vi "Serial Convert.vi"(8 "Range (V)":sgl=20.0 format="%#_13g", 10 "N channels bytes to read":u8=18, 11 "Raw serial buffer":string="\u0000\u0000\u0000\u0000\u0000\u0000\u0000\u0000\u0000\u0000\u0000\u0000\u0000\u0000\u0000\u0000\u0000\u0000") -> (0 "V6 (V)":sgl, 1 "V5 (V)":sgl, 2 "V4 (V)":sgl, 3 "V3 (V)":sgl, 4 "V7 (V)":sgl, 5 "V2 (V)":sgl, 6 "V8 (V)":sgl, 7 "V1 (V)":sgl)   [LabVIEW 2015]
panel:
  # "PN 19/12/2014, 17/08/2015 (nChan optimisation)"
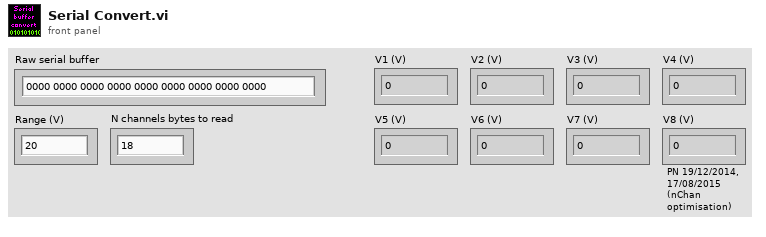
[diagram p1: front panel]
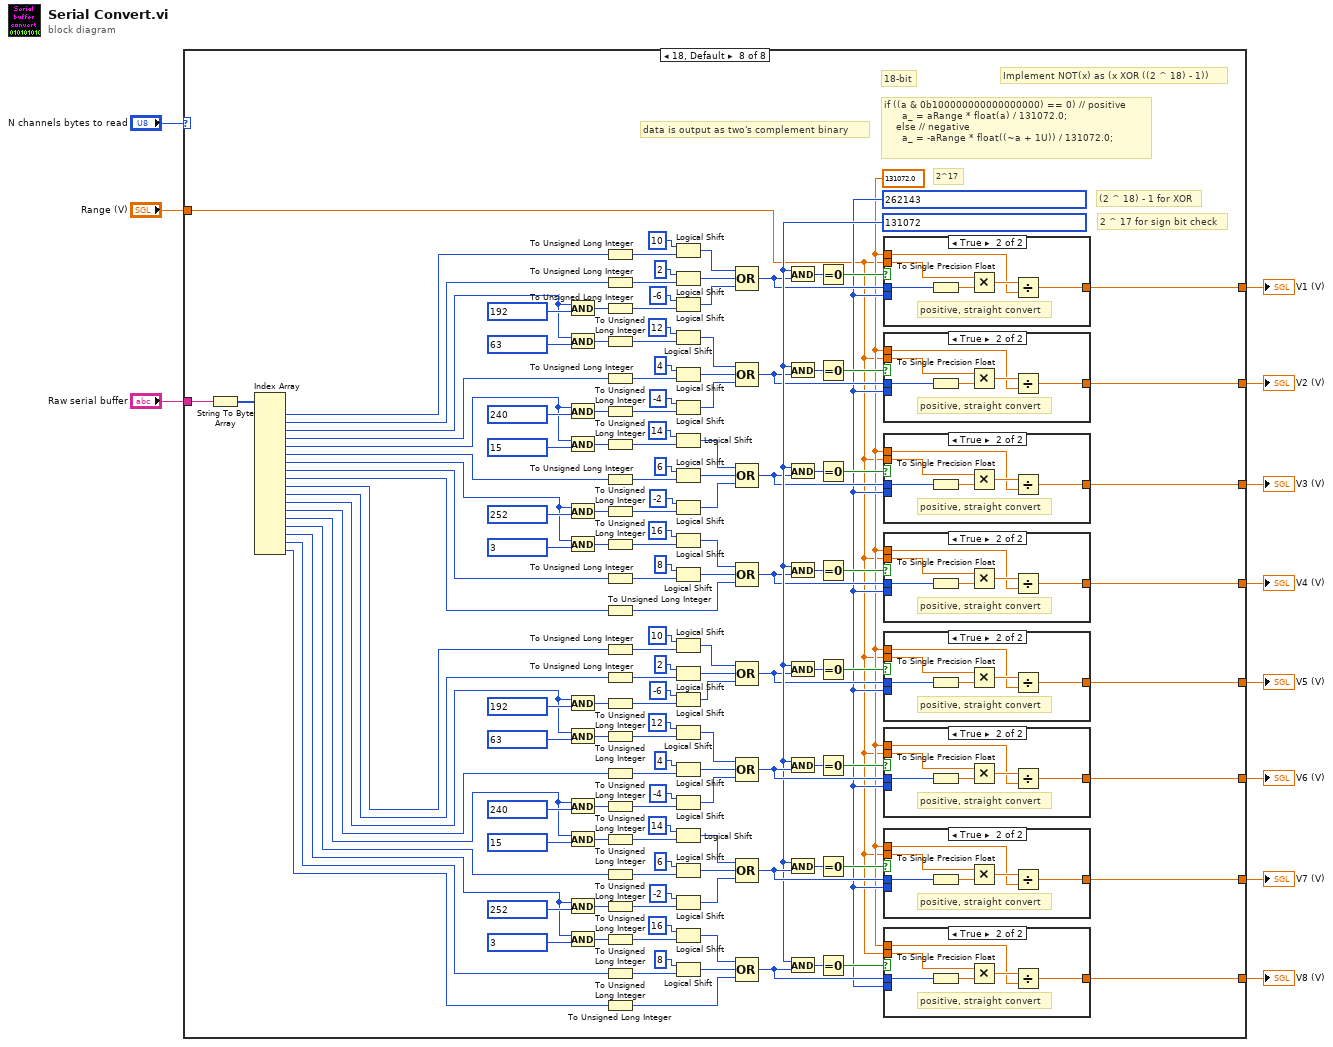
[diagram p0: block diagram]
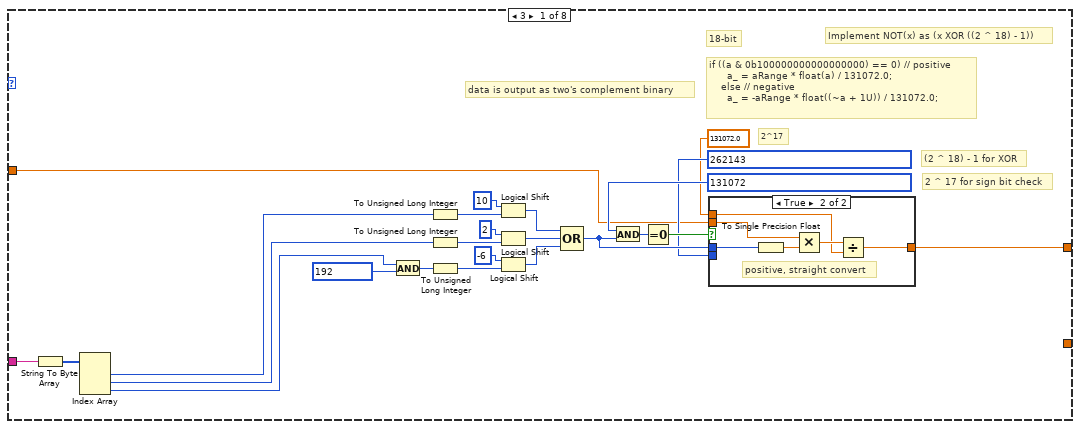
[diagram p2: hidden frame]
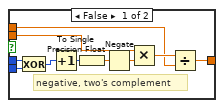
[diagram p3: hidden frame]
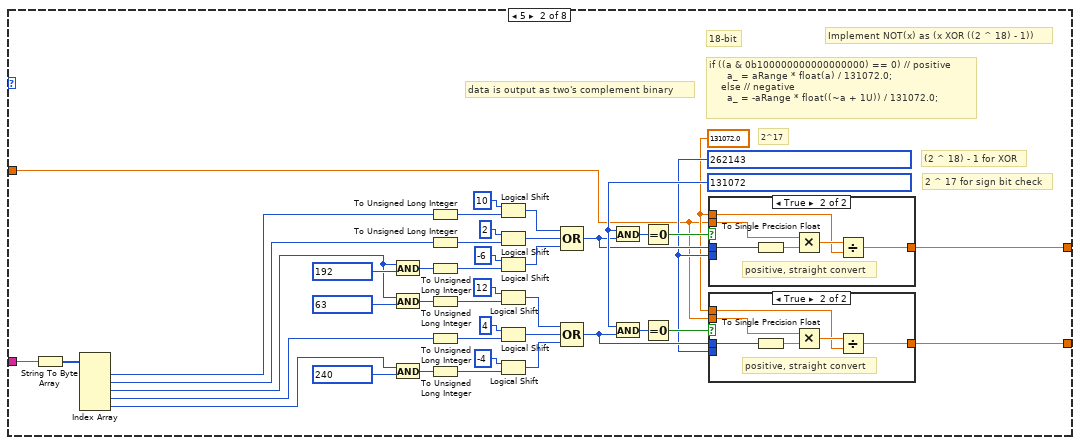
[diagram p4: hidden frame]
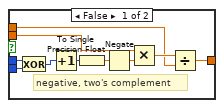
[diagram p5: hidden frame]
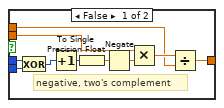
[diagram p6: hidden frame]
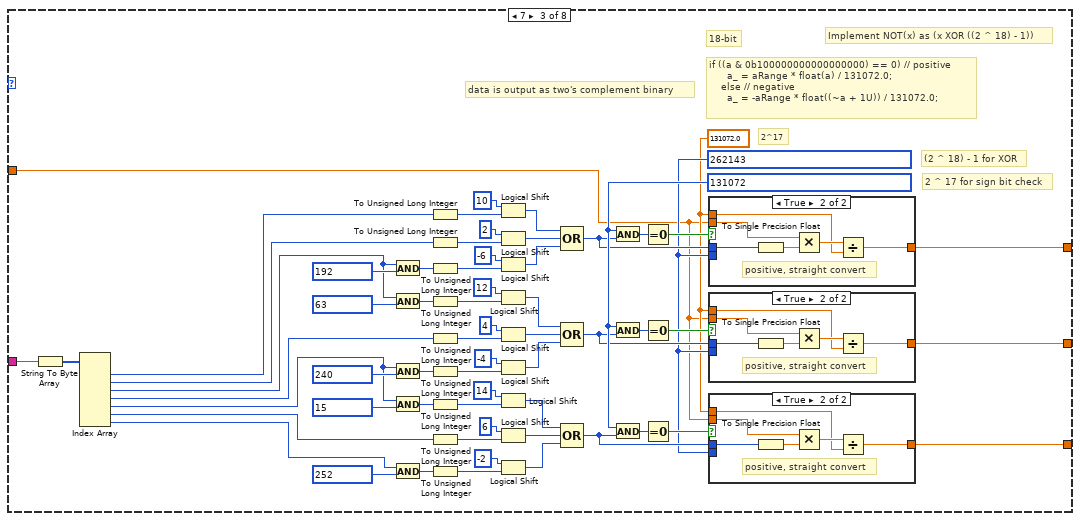
[diagram p7: hidden frame]
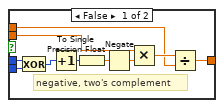
[diagram p8: hidden frame]
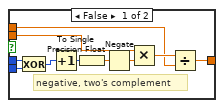
[diagram p9: hidden frame]
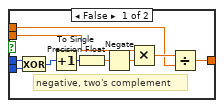
[diagram p10: hidden frame]
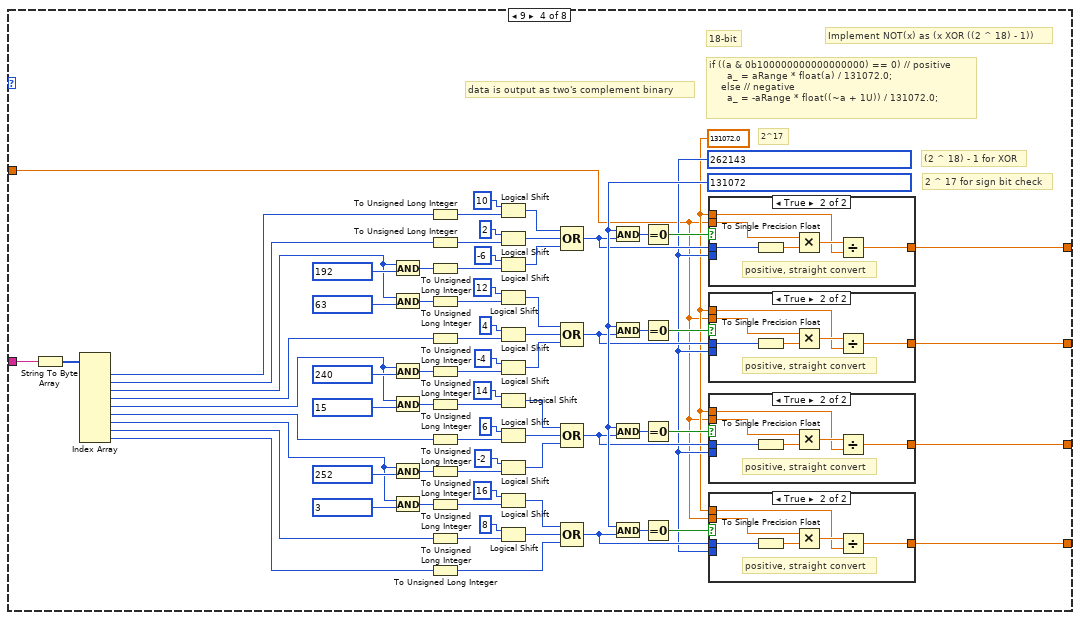
[diagram p11: hidden frame]
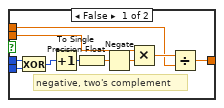
[diagram p12: hidden frame]
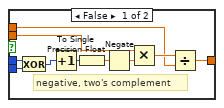
[diagram p13: hidden frame]
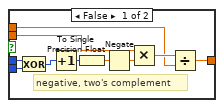
[diagram p14: hidden frame]
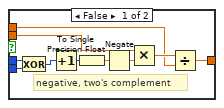
[diagram p15: hidden frame]
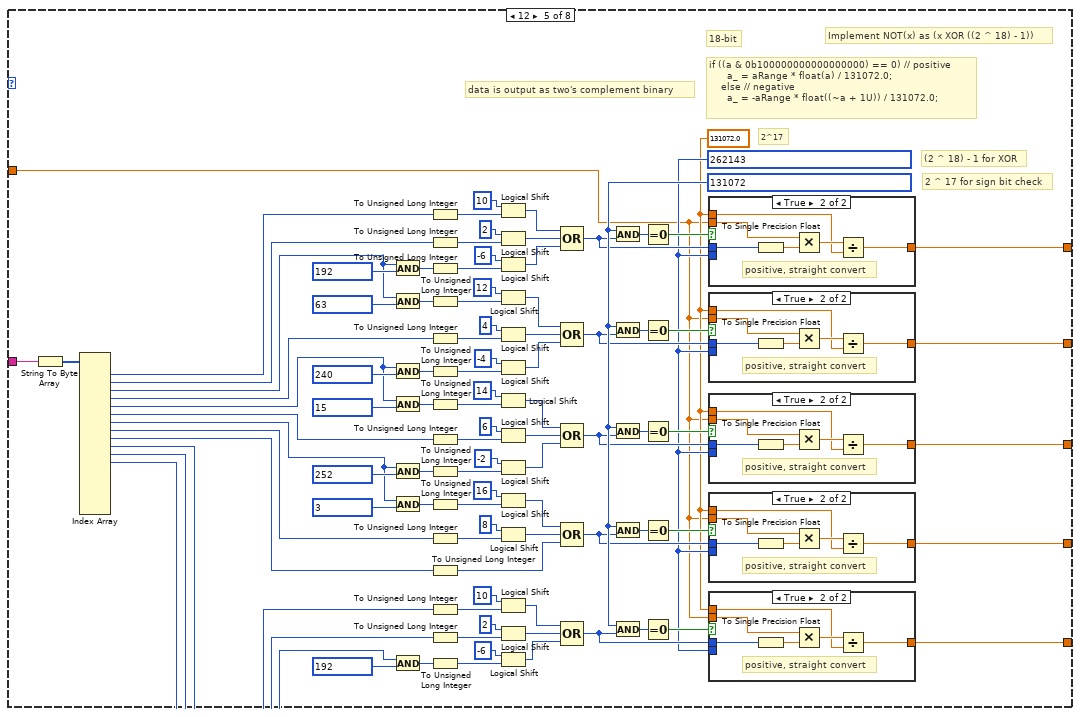
[diagram p16: hidden frame]
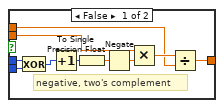
[diagram p17: hidden frame]
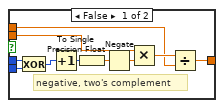
[diagram p18: hidden frame]
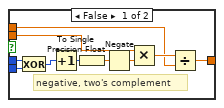
[diagram p19: hidden frame]
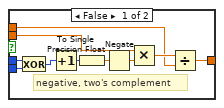
[diagram p20: hidden frame]
diagram:
  n1 = case shown="18, Default" "N channels bytes to read" {
    tunnel: "Raw serial buffer" -> [w35 w94 w188 w313 w472 w666 w895 w1155]
    tunnel: [_ _ _ _ _ _ w841 w1100] -> w10
    tunnel: [_ _ _ _ _ w613 w840 w1099] -> w9
    tunnel: [_ _ _ _ _ _ _ w1044] -> w8
    tunnel: [w20 w66 w147 w260 w407 w585 w798 w1043] -> w7
    tunnel: [_ _ w143 w256 w403 w581 w794 w1039] -> w6
    tunnel: [_ w63 w142 w255 w402 w580 w793 w1038] -> w5
    tunnel: [_ _ _ w254 w401 w579 w792 w1037] -> w4
    tunnel: [_ _ _ _ w400 w578 w791 w1036] -> w3
    tunnel: "Range (V)" -> [w15 w58 w136 w246 w390 w568 w781 w1026]
    frame 3 {
      # "2 ^ 17 for sign bit check"
      # "(2 ^ 18) - 1 for XOR"
      # "Implement NOT(x) as (x XOR ((2 ^ 18) - 1))"
      # "18-bit"
      # "2^17"
      # "data is output as two's complement binary"
      # "if ((a & 0b100000000000000000) == 0) // positive\n      a_ = aRange * float(a) / 131072.0; \n    else // negative\n      a_ = -aRange * float((~a + 1U)) / 131072.0;"
      n2 = String To Byte Array(string=w35) -> (unsigned byte array=w30:u8[])
      n3 = Index Array(array=w30) -> (element #1=w34:u8, element #2=w31:u8, element #3=w23:u8)  [unwired: 3 in]
      n4 = And(x=w23, y=u8 192) -> (x .and. y?=w26:u8)
      n5 = To Unsigned Long Integer(number=w34) -> (unsigned 32bit integer=w29:u32)
      n6 = To Unsigned Long Integer(number=w31) -> (unsigned 32bit integer=w28:u32)
      n7 = To Unsigned Long Integer(number=w26) -> (unsigned 32bit integer=w13:u32)
      n8 = Logical Shift(y=i16 10, x=w29) -> (x << y=w24:u32)
      n9 = Logical Shift(y=i16 2, x=w28) -> (x << y=w25:u32)
      n10 = Logical Shift(y=i16 -6, x=w13) -> (x << y=w12:u32)
      n11 = Compound Arithmetic op=OR(w24, w25, w12) -> (w18:u32)
      n12 = And(x=u32 131072, y=w18) -> (x .and. y?=w22:u32)
      n13 = Equal To 0?(x=w22) -> (x = 0?=w19:bool)
      n14 = case shown="True" w19 {
        tunnel: w15 -> [w42 w49]
        tunnel: sgl 131072.0 -> [w41 w47]
        tunnel: w18 -> [w37 w51]
        tunnel: [w40 w46] -> w20
        tunnel: u32 262143 -> [w36 _]
        frame False {
          # "negative, two's complement"
          n15 = Exclusive Or(1:w36, 2:w37) -> (0:w38:u32)
          n16 = Increment(x=w38) -> (x+1=w43:u32)
          n17 = To Single Precision Float(number=w43) -> (single precision float=w45:sgl)
          n18 = Negate(x=w45) -> (-x=w39:sgl)
          n19 = Multiply(x=w42, y=w39) -> (x*y=w44:sgl)
          n20 = Divide(x=w44, y=w41) -> (x/y=w40:sgl)
        }
        frame True {
          # "positive, straight convert"
          n21 = To Single Precision Float(number=w51) -> (single precision float=w50:sgl)
          n22 = Multiply(x=w49, y=w50) -> (x*y=w48:sgl)
          n23 = Divide(x=w48, y=w47) -> (x/y=w46:sgl)
        }
      }
    }
    frame 5 {
      w60 = u32 262143
      w59 = sgl 131072.0
      w67 = u32 131072
      # "2 ^ 17 for sign bit check"
      # "(2 ^ 18) - 1 for XOR"
      # "Implement NOT(x) as (x XOR ((2 ^ 18) - 1))"
      # "18-bit"
      # "2^17"
      # "data is output as two's complement binary"
      # "if ((a & 0b100000000000000000) == 0) // positive\n      a_ = aRange * float(a) / 131072.0; \n    else // negative\n      a_ = -aRange * float((~a + 1U)) / 131072.0;"
      n24 = String To Byte Array(string=w94) -> (unsigned byte array=w89:u8[])
      n25 = Index Array(array=w89) -> (element #1=w93:u8, element #2=w90:u8, element #3=w81:u8, element #4=w77:u8, element #5=w70:u8)  [unwired: 5 in]
      n26 = And(x=w81, y=u8 192) -> (x .and. y?=w85:u8)
      n27 = And(x=w81, y=u8 63) -> (x .and. y?=w80:u8)
      n28 = And(x=w70, y=u8 240) -> (x .and. y?=w73:u8)
      n29 = To Unsigned Long Integer(number=w93) -> (unsigned 32bit integer=w88:u32)
      n30 = To Unsigned Long Integer(number=w90) -> (unsigned 32bit integer=w87:u32)
      n31 = To Unsigned Long Integer(number=w85) -> (unsigned 32bit integer=w56:u32)
      n32 = To Unsigned Long Integer(number=w80) -> (unsigned 32bit integer=w79:u32)
      n33 = To Unsigned Long Integer(number=w77) -> (unsigned 32bit integer=w76:u32)
      n34 = To Unsigned Long Integer(number=w73) -> (unsigned 32bit integer=w53:u32)
      n35 = Logical Shift(y=i16 10, x=w88) -> (x << y=w83:u32)
      n36 = Logical Shift(y=i16 2, x=w87) -> (x << y=w84:u32)
      n37 = Logical Shift(y=i16 -6, x=w56) -> (x << y=w55:u32)
      n38 = Logical Shift(y=i16 12, x=w79) -> (x << y=w72:u32)
      n39 = Logical Shift(y=i16 4, x=w76) -> (x << y=w71:u32)
      n40 = Logical Shift(y=i16 -4, x=w53) -> (x << y=w52:u32)
      n41 = Compound Arithmetic op=OR(w83, w84, w55) -> (w64:u32)
      n42 = Compound Arithmetic op=OR(w72, w71, w52) -> (w61:u32)
      n43 = And(x=w67, y=w64) -> (x .and. y?=w69:u32)
      n44 = And(x=w67, y=w61) -> (x .and. y?=w68:u32)
      n45 = Equal To 0?(x=w69) -> (x = 0?=w65:bool)
      n46 = Equal To 0?(x=w68) -> (x = 0?=w62:bool)
      n47 = case shown="True" w65 {
        tunnel: w58 -> [w101 w108]
        tunnel: w59 -> [w100 w106]
        tunnel: w64 -> [w96 w110]
        tunnel: [w99 w105] -> w66
        tunnel: w60 -> [w95 _]
        frame False {
          # "negative, two's complement"
          n48 = Exclusive Or(1:w95, 2:w96) -> (0:w97:u32)
          n49 = Increment(x=w97) -> (x+1=w102:u32)
          n50 = To Single Precision Float(number=w102) -> (single precision float=w104:sgl)
          n51 = Negate(x=w104) -> (-x=w98:sgl)
          n52 = Multiply(x=w101, y=w98) -> (x*y=w103:sgl)
          n53 = Divide(x=w103, y=w100) -> (x/y=w99:sgl)
        }
        frame True {
          # "positive, straight convert"
          n54 = To Single Precision Float(number=w110) -> (single precision float=w109:sgl)
          n55 = Multiply(x=w108, y=w109) -> (x*y=w107:sgl)
          n56 = Divide(x=w107, y=w106) -> (x/y=w105:sgl)
        }
      }
      n57 = case shown="True" w62 {
        tunnel: w58 -> [w117 w124]
        tunnel: w59 -> [w116 w122]
        tunnel: w61 -> [w112 w126]
        tunnel: [w115 w121] -> w63
        tunnel: w60 -> [w111 _]
        frame False {
          # "negative, two's complement"
          n58 = Exclusive Or(1:w111, 2:w112) -> (0:w113:u32)
          n59 = Increment(x=w113) -> (x+1=w118:u32)
          n60 = To Single Precision Float(number=w118) -> (single precision float=w120:sgl)
          n61 = Negate(x=w120) -> (-x=w114:sgl)
          n62 = Multiply(x=w117, y=w114) -> (x*y=w119:sgl)
          n63 = Divide(x=w119, y=w116) -> (x/y=w115:sgl)
        }
        frame True {
          # "positive, straight convert"
          n64 = To Single Precision Float(number=w126) -> (single precision float=w125:sgl)
          n65 = Multiply(x=w124, y=w125) -> (x*y=w123:sgl)
          n66 = Divide(x=w123, y=w122) -> (x/y=w121:sgl)
        }
      }
    }
    frame 7 {
      w138 = u32 262143
      w137 = sgl 131072.0
      w148 = u32 131072
      # "2 ^ 17 for sign bit check"
      # "(2 ^ 18) - 1 for XOR"
      # "Implement NOT(x) as (x XOR ((2 ^ 18) - 1))"
      # "18-bit"
      # "2^17"
      # "data is output as two's complement binary"
      # "if ((a & 0b100000000000000000) == 0) // positive\n      a_ = aRange * float(a) / 131072.0; \n    else // negative\n      a_ = -aRange * float((~a + 1U)) / 131072.0;"
      n67 = String To Byte Array(string=w188) -> (unsigned byte array=w183:u8[])
      n68 = Index Array(array=w183) -> (element #1=w187:u8, element #2=w184:u8, element #3=w175:u8, element #4=w171:u8, element #5=w163:u8, element #6=w158:u8, element #7=w152:u8)  [unwired: 7 in]
      n69 = And(x=w175, y=u8 192) -> (x .and. y?=w179:u8)
      n70 = And(x=w175, y=u8 63) -> (x .and. y?=w174:u8)
      n71 = And(x=w163, y=u8 240) -> (x .and. y?=w167:u8)
      n72 = And(x=w163, y=u8 15) -> (x .and. y?=w162:u8)
      n73 = And(x=w152, y=u8 252) -> (x .and. y?=w153:u8)
      n74 = To Unsigned Long Integer(number=w187) -> (unsigned 32bit integer=w182:u32)
      n75 = To Unsigned Long Integer(number=w184) -> (unsigned 32bit integer=w181:u32)
      n76 = To Unsigned Long Integer(number=w179) -> (unsigned 32bit integer=w134:u32)
      n77 = To Unsigned Long Integer(number=w174) -> (unsigned 32bit integer=w173:u32)
      n78 = To Unsigned Long Integer(number=w171) -> (unsigned 32bit integer=w170:u32)
      n79 = To Unsigned Long Integer(number=w167) -> (unsigned 32bit integer=w131:u32)
      n80 = To Unsigned Long Integer(number=w162) -> (unsigned 32bit integer=w160:u32)
      n81 = To Unsigned Long Integer(number=w158) -> (unsigned 32bit integer=w156:u32)
      n82 = To Unsigned Long Integer(number=w153) -> (unsigned 32bit integer=w127:u32)
      n83 = Logical Shift(y=i16 10, x=w182) -> (x << y=w177:u32)
      n84 = Logical Shift(y=i16 2, x=w181) -> (x << y=w178:u32)
      n85 = Logical Shift(y=i16 -6, x=w134) -> (x << y=w133:u32)
      n86 = Logical Shift(y=i16 12, x=w173) -> (x << y=w166:u32)
      n87 = Logical Shift(y=i16 4, x=w170) -> (x << y=w165:u32)
      n88 = Logical Shift(y=i16 -4, x=w131) -> (x << y=w130:u32)
      n89 = Logical Shift(y=i16 14, x=w160) -> (x << y=w159:u32)
      n90 = Logical Shift(y=i16 6, x=w156) -> (x << y=w155:u32)
      n91 = Logical Shift(y=i16 -2, x=w127) -> (x << y=w128:u32)
      n92 = Compound Arithmetic op=OR(w177, w178, w133) -> (w145:u32)
      n93 = Compound Arithmetic op=OR(w166, w165, w130) -> (w139:u32)
      n94 = Compound Arithmetic op=OR(w159, w155, w128) -> (w141:u32)
      n95 = And(x=w148, y=w145) -> (x .and. y?=w151:u32)
      n96 = And(x=w148, y=w139) -> (x .and. y?=w150:u32)
      n97 = And(x=w148, y=w141) -> (x .and. y?=w149:u32)
      n98 = Equal To 0?(x=w151) -> (x = 0?=w146:bool)
      n99 = Equal To 0?(x=w150) -> (x = 0?=w140:bool)
      n100 = Equal To 0?(x=w149) -> (x = 0?=w144:bool)
      n101 = case shown="True" w146 {
        tunnel: w136 -> [w195 w202]
        tunnel: w137 -> [w194 w200]
        tunnel: w145 -> [w190 w204]
        tunnel: [w193 w199] -> w147
        tunnel: w138 -> [w189 _]
        frame False {
          # "negative, two's complement"
          n102 = Exclusive Or(1:w189, 2:w190) -> (0:w191:u32)
          n103 = Increment(x=w191) -> (x+1=w196:u32)
          n104 = To Single Precision Float(number=w196) -> (single precision float=w198:sgl)
          n105 = Negate(x=w198) -> (-x=w192:sgl)
          n106 = Multiply(x=w195, y=w192) -> (x*y=w197:sgl)
          n107 = Divide(x=w197, y=w194) -> (x/y=w193:sgl)
        }
        frame True {
          # "positive, straight convert"
          n108 = To Single Precision Float(number=w204) -> (single precision float=w203:sgl)
          n109 = Multiply(x=w202, y=w203) -> (x*y=w201:sgl)
          n110 = Divide(x=w201, y=w200) -> (x/y=w199:sgl)
        }
      }
      n111 = case shown="True" w140 {
        tunnel: w136 -> [w211 w218]
        tunnel: w137 -> [w210 w216]
        tunnel: w139 -> [w206 w220]
        tunnel: [w209 w215] -> w142
        tunnel: w138 -> [w205 _]
        frame False {
          # "negative, two's complement"
          n112 = Exclusive Or(1:w205, 2:w206) -> (0:w207:u32)
          n113 = Increment(x=w207) -> (x+1=w212:u32)
          n114 = To Single Precision Float(number=w212) -> (single precision float=w214:sgl)
          n115 = Negate(x=w214) -> (-x=w208:sgl)
          n116 = Multiply(x=w211, y=w208) -> (x*y=w213:sgl)
          n117 = Divide(x=w213, y=w210) -> (x/y=w209:sgl)
        }
        frame True {
          # "positive, straight convert"
          n118 = To Single Precision Float(number=w220) -> (single precision float=w219:sgl)
          n119 = Multiply(x=w218, y=w219) -> (x*y=w217:sgl)
          n120 = Divide(x=w217, y=w216) -> (x/y=w215:sgl)
        }
      }
      n121 = case shown="True" w144 {
        tunnel: w136 -> [w227 w234]
        tunnel: w137 -> [w226 w232]
        tunnel: w141 -> [w222 w236]
        tunnel: [w225 w231] -> w143
        tunnel: w138 -> [w221 _]
        frame False {
          # "negative, two's complement"
          n122 = Exclusive Or(1:w221, 2:w222) -> (0:w223:u32)
          n123 = Increment(x=w223) -> (x+1=w228:u32)
          n124 = To Single Precision Float(number=w228) -> (single precision float=w230:sgl)
          n125 = Negate(x=w230) -> (-x=w224:sgl)
          n126 = Multiply(x=w227, y=w224) -> (x*y=w229:sgl)
          n127 = Divide(x=w229, y=w226) -> (x/y=w225:sgl)
        }
        frame True {
          # "positive, straight convert"
          n128 = To Single Precision Float(number=w236) -> (single precision float=w235:sgl)
          n129 = Multiply(x=w234, y=w235) -> (x*y=w233:sgl)
          n130 = Divide(x=w233, y=w232) -> (x/y=w231:sgl)
        }
      }
    }
    frame 9 {
      w248 = u32 262143
      w247 = sgl 131072.0
      w261 = u32 131072
      # "2 ^ 17 for sign bit check"
      # "(2 ^ 18) - 1 for XOR"
      # "Implement NOT(x) as (x XOR ((2 ^ 18) - 1))"
      # "18-bit"
      # "2^17"
      # "data is output as two's complement binary"
      # "if ((a & 0b100000000000000000) == 0) // positive\n      a_ = aRange * float(a) / 131072.0; \n    else // negative\n      a_ = -aRange * float((~a + 1U)) / 131072.0;"
      n131 = String To Byte Array(string=w313) -> (unsigned byte array=w308:u8[])
      n132 = Index Array(array=w308) -> (element #1=w312:u8, element #2=w309:u8, element #3=w300:u8, element #4=w296:u8, element #5=w288:u8, element #6=w283:u8, element #7=w276:u8, element #8=w271:u8, element #9=w267:u8)  [unwired: 9 in]
      n133 = And(x=w300, y=u8 192) -> (x .and. y?=w304:u8)
      n134 = And(x=w300, y=u8 63) -> (x .and. y?=w299:u8)
      n135 = And(x=w288, y=u8 240) -> (x .and. y?=w292:u8)
      n136 = And(x=w288, y=u8 15) -> (x .and. y?=w287:u8)
      n137 = And(x=w276, y=u8 252) -> (x .and. y?=w278:u8)
      n138 = And(x=w276, y=u8 3) -> (x .and. y?=w275:u8)
      n139 = To Unsigned Long Integer(number=w312) -> (unsigned 32bit integer=w307:u32)
      n140 = To Unsigned Long Integer(number=w309) -> (unsigned 32bit integer=w306:u32)
      n141 = To Unsigned Long Integer(number=w304) -> (unsigned 32bit integer=w244:u32)
      n142 = To Unsigned Long Integer(number=w299) -> (unsigned 32bit integer=w298:u32)
      n143 = To Unsigned Long Integer(number=w296) -> (unsigned 32bit integer=w295:u32)
      n144 = To Unsigned Long Integer(number=w292) -> (unsigned 32bit integer=w241:u32)
      n145 = To Unsigned Long Integer(number=w287) -> (unsigned 32bit integer=w285:u32)
      n146 = To Unsigned Long Integer(number=w283) -> (unsigned 32bit integer=w281:u32)
      n147 = To Unsigned Long Integer(number=w278) -> (unsigned 32bit integer=w237:u32)
      n148 = To Unsigned Long Integer(number=w275) -> (unsigned 32bit integer=w273:u32)
      n149 = To Unsigned Long Integer(number=w271) -> (unsigned 32bit integer=w269:u32)
      n150 = To Unsigned Long Integer(number=w267) -> (unsigned 32bit integer=w266:u32)
      n151 = Logical Shift(y=i16 10, x=w307) -> (x << y=w302:u32)
      n152 = Logical Shift(y=i16 2, x=w306) -> (x << y=w303:u32)
      n153 = Logical Shift(y=i16 -6, x=w244) -> (x << y=w243:u32)
      n154 = Logical Shift(y=i16 12, x=w298) -> (x << y=w291:u32)
      n155 = Logical Shift(y=i16 4, x=w295) -> (x << y=w290:u32)
      n156 = Logical Shift(y=i16 -4, x=w241) -> (x << y=w240:u32)
      n157 = Logical Shift(y=i16 14, x=w285) -> (x << y=w284:u32)
      n158 = Logical Shift(y=i16 6, x=w281) -> (x << y=w280:u32)
      n159 = Logical Shift(y=i16 -2, x=w237) -> (x << y=w238:u32)
      n160 = Logical Shift(y=i16 16, x=w273) -> (x << y=w272:u32)
      n161 = Logical Shift(y=i16 8, x=w269) -> (x << y=w268:u32)
      n162 = Compound Arithmetic op=OR(w302, w303, w243) -> (w258:u32)
      n163 = Compound Arithmetic op=OR(w291, w290, w240) -> (w249:u32)
      n164 = Compound Arithmetic op=OR(w284, w280, w238) -> (w252:u32)
      n165 = Compound Arithmetic op=OR(w272, w268, w266) -> (w251:u32)
      n166 = And(x=w261, y=w258) -> (x .and. y?=w265:u32)
      n167 = And(x=w261, y=w249) -> (x .and. y?=w264:u32)
      n168 = And(x=w261, y=w252) -> (x .and. y?=w263:u32)
      n169 = And(x=w261, y=w251) -> (x .and. y?=w262:u32)
      n170 = Equal To 0?(x=w265) -> (x = 0?=w259:bool)
      n171 = Equal To 0?(x=w264) -> (x = 0?=w250:bool)
      n172 = Equal To 0?(x=w263) -> (x = 0?=w257:bool)
      n173 = Equal To 0?(x=w262) -> (x = 0?=w253:bool)
      n174 = case shown="True" w259 {
        tunnel: w246 -> [w320 w327]
        tunnel: w247 -> [w319 w325]
        tunnel: w258 -> [w315 w329]
        tunnel: [w318 w324] -> w260
        tunnel: w248 -> [w314 _]
        frame False {
          # "negative, two's complement"
          n175 = Exclusive Or(1:w314, 2:w315) -> (0:w316:u32)
          n176 = Increment(x=w316) -> (x+1=w321:u32)
          n177 = To Single Precision Float(number=w321) -> (single precision float=w323:sgl)
          n178 = Negate(x=w323) -> (-x=w317:sgl)
          n179 = Multiply(x=w320, y=w317) -> (x*y=w322:sgl)
          n180 = Divide(x=w322, y=w319) -> (x/y=w318:sgl)
        }
        frame True {
          # "positive, straight convert"
          n181 = To Single Precision Float(number=w329) -> (single precision float=w328:sgl)
          n182 = Multiply(x=w327, y=w328) -> (x*y=w326:sgl)
          n183 = Divide(x=w326, y=w325) -> (x/y=w324:sgl)
        }
      }
      n184 = case shown="True" w250 {
        tunnel: w246 -> [w336 w343]
        tunnel: w247 -> [w335 w341]
        tunnel: w249 -> [w331 w345]
        tunnel: [w334 w340] -> w255
        tunnel: w248 -> [w330 _]
        frame False {
          # "negative, two's complement"
          n185 = Exclusive Or(1:w330, 2:w331) -> (0:w332:u32)
          n186 = Increment(x=w332) -> (x+1=w337:u32)
          n187 = To Single Precision Float(number=w337) -> (single precision float=w339:sgl)
          n188 = Negate(x=w339) -> (-x=w333:sgl)
          n189 = Multiply(x=w336, y=w333) -> (x*y=w338:sgl)
          n190 = Divide(x=w338, y=w335) -> (x/y=w334:sgl)
        }
        frame True {
          # "positive, straight convert"
          n191 = To Single Precision Float(number=w345) -> (single precision float=w344:sgl)
          n192 = Multiply(x=w343, y=w344) -> (x*y=w342:sgl)
          n193 = Divide(x=w342, y=w341) -> (x/y=w340:sgl)
        }
      }
      n194 = case shown="True" w257 {
        tunnel: w246 -> [w352 w359]
        tunnel: w247 -> [w351 w357]
        tunnel: w252 -> [w347 w361]
        tunnel: [w350 w356] -> w256
        tunnel: w248 -> [w346 _]
        frame False {
          # "negative, two's complement"
          n195 = Exclusive Or(1:w346, 2:w347) -> (0:w348:u32)
          n196 = Increment(x=w348) -> (x+1=w353:u32)
          n197 = To Single Precision Float(number=w353) -> (single precision float=w355:sgl)
          n198 = Negate(x=w355) -> (-x=w349:sgl)
          n199 = Multiply(x=w352, y=w349) -> (x*y=w354:sgl)
          n200 = Divide(x=w354, y=w351) -> (x/y=w350:sgl)
        }
        frame True {
          # "positive, straight convert"
          n201 = To Single Precision Float(number=w361) -> (single precision float=w360:sgl)
          n202 = Multiply(x=w359, y=w360) -> (x*y=w358:sgl)
          n203 = Divide(x=w358, y=w357) -> (x/y=w356:sgl)
        }
      }
      n204 = case shown="True" w253 {
        tunnel: w246 -> [w368 w375]
        tunnel: w247 -> [w367 w373]
        tunnel: w251 -> [w363 w377]
        tunnel: [w366 w372] -> w254
        tunnel: w248 -> [w362 _]
        frame False {
          # "negative, two's complement"
          n205 = Exclusive Or(1:w362, 2:w363) -> (0:w364:u32)
          n206 = Increment(x=w364) -> (x+1=w369:u32)
          n207 = To Single Precision Float(number=w369) -> (single precision float=w371:sgl)
          n208 = Negate(x=w371) -> (-x=w365:sgl)
          n209 = Multiply(x=w368, y=w365) -> (x*y=w370:sgl)
          n210 = Divide(x=w370, y=w367) -> (x/y=w366:sgl)
        }
        frame True {
          # "positive, straight convert"
          n211 = To Single Precision Float(number=w377) -> (single precision float=w376:sgl)
          n212 = Multiply(x=w375, y=w376) -> (x*y=w374:sgl)
          n213 = Divide(x=w374, y=w373) -> (x/y=w372:sgl)
        }
      }
    }
    frame 12 {
      w392 = u32 262143
      w391 = sgl 131072.0
      w411 = u32 131072
      # "2 ^ 17 for sign bit check"
      # "(2 ^ 18) - 1 for XOR"
      # "Implement NOT(x) as (x XOR ((2 ^ 18) - 1))"
      # "18-bit"
      # "2^17"
      # "data is output as two's complement binary"
      # "if ((a & 0b100000000000000000) == 0) // positive\n      a_ = aRange * float(a) / 131072.0; \n    else // negative\n      a_ = -aRange * float((~a + 1U)) / 131072.0;"
      n214 = String To Byte Array(string=w472) -> (unsigned byte array=w467:u8[])
      n215 = Index Array(array=w467) -> (element #1=w471:u8, element #2=w468:u8, element #3=w459:u8, element #4=w455:u8, element #5=w447:u8, element #6=w442:u8, element #7=w435:u8, element #8=w430:u8, element #9=w426:u8, element #10=w410:u8, element #11=w409:u8, element #12=w408:u8)  [unwired: 18 in, 6 out]
      n216 = And(x=w459, y=u8 192) -> (x .and. y?=w463:u8)
      n217 = And(x=w459, y=u8 63) -> (x .and. y?=w458:u8)
      n218 = And(x=w447, y=u8 240) -> (x .and. y?=w451:u8)
      n219 = And(x=w447, y=u8 15) -> (x .and. y?=w446:u8)
      n220 = And(x=w435, y=u8 252) -> (x .and. y?=w437:u8)
      n221 = And(x=w435, y=u8 3) -> (x .and. y?=w434:u8)
      n222 = And(x=w408, y=u8 192) -> (x .and. y?=w417:u8)
      n223 = To Unsigned Long Integer(number=w471) -> (unsigned 32bit integer=w466:u32)
      n224 = To Unsigned Long Integer(number=w468) -> (unsigned 32bit integer=w465:u32)
      n225 = To Unsigned Long Integer(number=w463) -> (unsigned 32bit integer=w388:u32)
      n226 = To Unsigned Long Integer(number=w458) -> (unsigned 32bit integer=w457:u32)
      n227 = To Unsigned Long Integer(number=w455) -> (unsigned 32bit integer=w454:u32)
      n228 = To Unsigned Long Integer(number=w451) -> (unsigned 32bit integer=w382:u32)
      n229 = To Unsigned Long Integer(number=w446) -> (unsigned 32bit integer=w444:u32)
      n230 = To Unsigned Long Integer(number=w442) -> (unsigned 32bit integer=w440:u32)
      n231 = To Unsigned Long Integer(number=w437) -> (unsigned 32bit integer=w378:u32)
      n232 = To Unsigned Long Integer(number=w434) -> (unsigned 32bit integer=w432:u32)
      n233 = To Unsigned Long Integer(number=w430) -> (unsigned 32bit integer=w428:u32)
      n234 = To Unsigned Long Integer(number=w426) -> (unsigned 32bit integer=w425:u32)
      n235 = To Unsigned Long Integer(number=w410) -> (unsigned 32bit integer=w414:u32)
      n236 = To Unsigned Long Integer(number=w409) -> (unsigned 32bit integer=w415:u32)
      n237 = To Unsigned Long Integer(number=w417) -> (unsigned 32bit integer=w384:u32)
      n238 = Logical Shift(y=i16 10, x=w466) -> (x << y=w461:u32)
      n239 = Logical Shift(y=i16 2, x=w465) -> (x << y=w462:u32)
      n240 = Logical Shift(y=i16 -6, x=w388) -> (x << y=w387:u32)
      n241 = Logical Shift(y=i16 12, x=w457) -> (x << y=w450:u32)
      n242 = Logical Shift(y=i16 4, x=w454) -> (x << y=w449:u32)
      n243 = Logical Shift(y=i16 -4, x=w382) -> (x << y=w381:u32)
      n244 = Logical Shift(y=i16 14, x=w444) -> (x << y=w443:u32)
      n245 = Logical Shift(y=i16 6, x=w440) -> (x << y=w439:u32)
      n246 = Logical Shift(y=i16 -2, x=w378) -> (x << y=w379:u32)
      n247 = Logical Shift(y=i16 16, x=w432) -> (x << y=w431:u32)
      n248 = Logical Shift(y=i16 8, x=w428) -> (x << y=w427:u32)
      n249 = Logical Shift(y=i16 10, x=w414) -> (x << y=w419:u32)
      n250 = Logical Shift(y=i16 2, x=w415) -> (x << y=w418:u32)
      n251 = Logical Shift(y=i16 -6, x=w384) -> (x << y=w385:u32)
      n252 = Compound Arithmetic op=OR(w461, w462, w387) -> (w405:u32)
      n253 = Compound Arithmetic op=OR(w450, w449, w381) -> (w394:u32)
      n254 = Compound Arithmetic op=OR(w443, w439, w379) -> (w397:u32)
      n255 = Compound Arithmetic op=OR(w431, w427, w425) -> (w396:u32)
      n256 = Compound Arithmetic op=OR(w419, w418, w385) -> (w393:u32)
      n257 = And(x=w411, y=w405) -> (x .and. y?=w424:u32)
      n258 = And(x=w411, y=w394) -> (x .and. y?=w423:u32)
      n259 = And(x=w411, y=w397) -> (x .and. y?=w422:u32)
      n260 = And(x=w411, y=w396) -> (x .and. y?=w421:u32)
      n261 = And(x=w411, y=w393) -> (x .and. y?=w420:u32)
      n262 = Equal To 0?(x=w424) -> (x = 0?=w406:bool)
      n263 = Equal To 0?(x=w423) -> (x = 0?=w395:bool)
      n264 = Equal To 0?(x=w422) -> (x = 0?=w404:bool)
      n265 = Equal To 0?(x=w421) -> (x = 0?=w399:bool)
      n266 = Equal To 0?(x=w420) -> (x = 0?=w398:bool)
      n267 = case shown="True" w406 {
        tunnel: w390 -> [w479 w486]
        tunnel: w391 -> [w478 w484]
        tunnel: w405 -> [w474 w488]
        tunnel: [w477 w483] -> w407
        tunnel: w392 -> [w473 _]
        frame False {
          # "negative, two's complement"
          n268 = Exclusive Or(1:w473, 2:w474) -> (0:w475:u32)
          n269 = Increment(x=w475) -> (x+1=w480:u32)
          n270 = To Single Precision Float(number=w480) -> (single precision float=w482:sgl)
          n271 = Negate(x=w482) -> (-x=w476:sgl)
          n272 = Multiply(x=w479, y=w476) -> (x*y=w481:sgl)
          n273 = Divide(x=w481, y=w478) -> (x/y=w477:sgl)
        }
        frame True {
          # "positive, straight convert"
          n274 = To Single Precision Float(number=w488) -> (single precision float=w487:sgl)
          n275 = Multiply(x=w486, y=w487) -> (x*y=w485:sgl)
          n276 = Divide(x=w485, y=w484) -> (x/y=w483:sgl)
        }
      }
      n277 = case shown="True" w395 {
        tunnel: w390 -> [w495 w502]
        tunnel: w391 -> [w494 w500]
        tunnel: w394 -> [w490 w504]
        tunnel: [w493 w499] -> w402
        tunnel: w392 -> [w489 _]
        frame False {
          # "negative, two's complement"
          n278 = Exclusive Or(1:w489, 2:w490) -> (0:w491:u32)
          n279 = Increment(x=w491) -> (x+1=w496:u32)
          n280 = To Single Precision Float(number=w496) -> (single precision float=w498:sgl)
          n281 = Negate(x=w498) -> (-x=w492:sgl)
          n282 = Multiply(x=w495, y=w492) -> (x*y=w497:sgl)
          n283 = Divide(x=w497, y=w494) -> (x/y=w493:sgl)
        }
        frame True {
          # "positive, straight convert"
          n284 = To Single Precision Float(number=w504) -> (single precision float=w503:sgl)
          n285 = Multiply(x=w502, y=w503) -> (x*y=w501:sgl)
          n286 = Divide(x=w501, y=w500) -> (x/y=w499:sgl)
        }
      }
      n287 = case shown="True" w404 {
        tunnel: w390 -> [w511 w518]
        tunnel: w391 -> [w510 w516]
        tunnel: w397 -> [w506 w520]
        tunnel: [w509 w515] -> w403
        tunnel: w392 -> [w505 _]
        frame False {
          # "negative, two's complement"
          n288 = Exclusive Or(1:w505, 2:w506) -> (0:w507:u32)
          n289 = Increment(x=w507) -> (x+1=w512:u32)
          n290 = To Single Precision Float(number=w512) -> (single precision float=w514:sgl)
          n291 = Negate(x=w514) -> (-x=w508:sgl)
          n292 = Multiply(x=w511, y=w508) -> (x*y=w513:sgl)
          n293 = Divide(x=w513, y=w510) -> (x/y=w509:sgl)
        }
        frame True {
          # "positive, straight convert"
          n294 = To Single Precision Float(number=w520) -> (single precision float=w519:sgl)
          n295 = Multiply(x=w518, y=w519) -> (x*y=w517:sgl)
          n296 = Divide(x=w517, y=w516) -> (x/y=w515:sgl)
        }
      }
      n297 = case shown="True" w399 {
        tunnel: w390 -> [w527 w534]
        tunnel: w391 -> [w526 w532]
        tunnel: w396 -> [w522 w536]
        tunnel: [w525 w531] -> w401
        tunnel: w392 -> [w521 _]
        frame False {
          # "negative, two's complement"
          n298 = Exclusive Or(1:w521, 2:w522) -> (0:w523:u32)
          n299 = Increment(x=w523) -> (x+1=w528:u32)
          n300 = To Single Precision Float(number=w528) -> (single precision float=w530:sgl)
          n301 = Negate(x=w530) -> (-x=w524:sgl)
          n302 = Multiply(x=w527, y=w524) -> (x*y=w529:sgl)
          n303 = Divide(x=w529, y=w526) -> (x/y=w525:sgl)
        }
        frame True {
          # "positive, straight convert"
          n304 = To Single Precision Float(number=w536) -> (single precision float=w535:sgl)
          n305 = Multiply(x=w534, y=w535) -> (x*y=w533:sgl)
          n306 = Divide(x=w533, y=w532) -> (x/y=w531:sgl)
        }
      }
      n307 = case shown="True" w398 {
        tunnel: w390 -> [w543 w550]
        tunnel: w391 -> [w542 w548]
        tunnel: w393 -> [w538 w552]
        tunnel: [w541 w547] -> w400
        tunnel: w392 -> [w537 _]
        frame False {
          # "negative, two's complement"
          n308 = Exclusive Or(1:w537, 2:w538) -> (0:w539:u32)
          n309 = Increment(x=w539) -> (x+1=w544:u32)
          n310 = To Single Precision Float(number=w544) -> (single precision float=w546:sgl)
          n311 = Negate(x=w546) -> (-x=w540:sgl)
          n312 = Multiply(x=w543, y=w540) -> (x*y=w545:sgl)
          n313 = Divide(x=w545, y=w542) -> (x/y=w541:sgl)
        }
        frame True {
          # "positive, straight convert"
          n314 = To Single Precision Float(number=w552) -> (single precision float=w551:sgl)
          n315 = Multiply(x=w550, y=w551) -> (x*y=w549:sgl)
          n316 = Divide(x=w549, y=w548) -> (x/y=w547:sgl)
        }
      }
    }
    frame 14 {
      w570 = u32 262143
      w569 = sgl 131072.0
      w591 = u32 131072
      # "2 ^ 17 for sign bit check"
      # "(2 ^ 18) - 1 for XOR"
      # "Implement NOT(x) as (x XOR ((2 ^ 18) - 1))"
      # "18-bit"
      # "2^17"
      # "data is output as two's complement binary"
      # "if ((a & 0b100000000000000000) == 0) // positive\n      a_ = aRange * float(a) / 131072.0; \n    else // negative\n      a_ = -aRange * float((~a + 1U)) / 131072.0;"
      n317 = String To Byte Array(string=w666) -> (unsigned byte array=w661:u8[])
      n318 = Index Array(array=w661) -> (element #1=w665:u8, element #2=w662:u8, element #3=w653:u8, element #4=w649:u8, element #5=w641:u8, element #6=w636:u8, element #7=w629:u8, element #8=w624:u8, element #9=w620:u8, element #10=w590:u8, element #11=w589:u8, element #12=w588:u8, element #13=w587:u8, element #14=w586:u8)  [unwired: 18 in, 4 out]
      n319 = And(x=w653, y=u8 192) -> (x .and. y?=w657:u8)
      n320 = And(x=w653, y=u8 63) -> (x .and. y?=w652:u8)
      n321 = And(x=w641, y=u8 240) -> (x .and. y?=w645:u8)
      n322 = And(x=w641, y=u8 15) -> (x .and. y?=w640:u8)
      n323 = And(x=w629, y=u8 252) -> (x .and. y?=w631:u8)
      n324 = And(x=w629, y=u8 3) -> (x .and. y?=w628:u8)
      n325 = And(x=w588, y=u8 192) -> (x .and. y?=w597:u8)
      n326 = And(x=w588, y=u8 63) -> (x .and. y?=w601:u8)
      n327 = And(x=w586, y=u8 240) -> (x .and. y?=w607:u8)
      n328 = To Unsigned Long Integer(number=w665) -> (unsigned 32bit integer=w660:u32)
      n329 = To Unsigned Long Integer(number=w662) -> (unsigned 32bit integer=w659:u32)
      n330 = To Unsigned Long Integer(number=w657) -> (unsigned 32bit integer=w566:u32)
      n331 = To Unsigned Long Integer(number=w652) -> (unsigned 32bit integer=w651:u32)
      n332 = To Unsigned Long Integer(number=w649) -> (unsigned 32bit integer=w648:u32)
      n333 = To Unsigned Long Integer(number=w645) -> (unsigned 32bit integer=w560:u32)
      n334 = To Unsigned Long Integer(number=w640) -> (unsigned 32bit integer=w638:u32)
      n335 = To Unsigned Long Integer(number=w636) -> (unsigned 32bit integer=w634:u32)
      n336 = To Unsigned Long Integer(number=w631) -> (unsigned 32bit integer=w556:u32)
      n337 = To Unsigned Long Integer(number=w628) -> (unsigned 32bit integer=w626:u32)
      n338 = To Unsigned Long Integer(number=w624) -> (unsigned 32bit integer=w622:u32)
      n339 = To Unsigned Long Integer(number=w620) -> (unsigned 32bit integer=w619:u32)
      n340 = To Unsigned Long Integer(number=w590) -> (unsigned 32bit integer=w594:u32)
      n341 = To Unsigned Long Integer(number=w589) -> (unsigned 32bit integer=w595:u32)
      n342 = To Unsigned Long Integer(number=w597) -> (unsigned 32bit integer=w562:u32)
      n343 = To Unsigned Long Integer(number=w601) -> (unsigned 32bit integer=w602:u32)
      n344 = To Unsigned Long Integer(number=w587) -> (unsigned 32bit integer=w604:u32)
      n345 = To Unsigned Long Integer(number=w607) -> (unsigned 32bit integer=w554:u32)
      n346 = Logical Shift(y=i16 10, x=w660) -> (x << y=w655:u32)
      n347 = Logical Shift(y=i16 2, x=w659) -> (x << y=w656:u32)
      n348 = Logical Shift(y=i16 -6, x=w566) -> (x << y=w565:u32)
      n349 = Logical Shift(y=i16 12, x=w651) -> (x << y=w644:u32)
      n350 = Logical Shift(y=i16 4, x=w648) -> (x << y=w643:u32)
      n351 = Logical Shift(y=i16 -4, x=w560) -> (x << y=w559:u32)
      n352 = Logical Shift(y=i16 14, x=w638) -> (x << y=w637:u32)
      n353 = Logical Shift(y=i16 6, x=w634) -> (x << y=w633:u32)
      n354 = Logical Shift(y=i16 -2, x=w556) -> (x << y=w557:u32)
      n355 = Logical Shift(y=i16 16, x=w626) -> (x << y=w625:u32)
      n356 = Logical Shift(y=i16 8, x=w622) -> (x << y=w621:u32)
      n357 = Logical Shift(y=i16 10, x=w594) -> (x << y=w599:u32)
      n358 = Logical Shift(y=i16 2, x=w595) -> (x << y=w598:u32)
      n359 = Logical Shift(y=i16 -6, x=w562) -> (x << y=w563:u32)
      n360 = Logical Shift(y=i16 12, x=w602) -> (x << y=w608:u32)
      n361 = Logical Shift(y=i16 4, x=w604) -> (x << y=w609:u32)
      n362 = Logical Shift(y=i16 -4, x=w554) -> (x << y=w553:u32)
      n363 = Compound Arithmetic op=OR(w655, w656, w565) -> (w583:u32)
      n364 = Compound Arithmetic op=OR(w644, w643, w559) -> (w572:u32)
      n365 = Compound Arithmetic op=OR(w637, w633, w557) -> (w575:u32)
      n366 = Compound Arithmetic op=OR(w625, w621, w619) -> (w574:u32)
      n367 = Compound Arithmetic op=OR(w599, w598, w563) -> (w571:u32)
      n368 = Compound Arithmetic op=OR(w608, w609, w553) -> (w614:u32)
      n369 = And(x=w591, y=w583) -> (x .and. y?=w618:u32)
      n370 = And(x=w591, y=w572) -> (x .and. y?=w617:u32)
      n371 = And(x=w591, y=w575) -> (x .and. y?=w616:u32)
      n372 = And(x=w591, y=w574) -> (x .and. y?=w615:u32)
      n373 = And(x=w591, y=w571) -> (x .and. y?=w610:u32)
      n374 = And(x=w591, y=w614) -> (x .and. y?=w611:u32)
      n375 = Equal To 0?(x=w618) -> (x = 0?=w584:bool)
      n376 = Equal To 0?(x=w617) -> (x = 0?=w573:bool)
      n377 = Equal To 0?(x=w616) -> (x = 0?=w582:bool)
      n378 = Equal To 0?(x=w615) -> (x = 0?=w577:bool)
      n379 = Equal To 0?(x=w610) -> (x = 0?=w576:bool)
      n380 = Equal To 0?(x=w611) -> (x = 0?=w612:bool)
      n381 = case shown="True" w584 {
        tunnel: w568 -> [w673 w680]
        tunnel: w569 -> [w672 w678]
        tunnel: w583 -> [w668 w682]
        tunnel: [w671 w677] -> w585
        tunnel: w570 -> [w667 _]
        frame False {
          # "negative, two's complement"
          n382 = Exclusive Or(1:w667, 2:w668) -> (0:w669:u32)
          n383 = Increment(x=w669) -> (x+1=w674:u32)
          n384 = To Single Precision Float(number=w674) -> (single precision float=w676:sgl)
          n385 = Negate(x=w676) -> (-x=w670:sgl)
          n386 = Multiply(x=w673, y=w670) -> (x*y=w675:sgl)
          n387 = Divide(x=w675, y=w672) -> (x/y=w671:sgl)
        }
        frame True {
          # "positive, straight convert"
          n388 = To Single Precision Float(number=w682) -> (single precision float=w681:sgl)
          n389 = Multiply(x=w680, y=w681) -> (x*y=w679:sgl)
          n390 = Divide(x=w679, y=w678) -> (x/y=w677:sgl)
        }
      }
      n391 = case shown="True" w573 {
        tunnel: w568 -> [w689 w696]
        tunnel: w569 -> [w688 w694]
        tunnel: w572 -> [w684 w698]
        tunnel: [w687 w693] -> w580
        tunnel: w570 -> [w683 _]
        frame False {
          # "negative, two's complement"
          n392 = Exclusive Or(1:w683, 2:w684) -> (0:w685:u32)
          n393 = Increment(x=w685) -> (x+1=w690:u32)
          n394 = To Single Precision Float(number=w690) -> (single precision float=w692:sgl)
          n395 = Negate(x=w692) -> (-x=w686:sgl)
          n396 = Multiply(x=w689, y=w686) -> (x*y=w691:sgl)
          n397 = Divide(x=w691, y=w688) -> (x/y=w687:sgl)
        }
        frame True {
          # "positive, straight convert"
          n398 = To Single Precision Float(number=w698) -> (single precision float=w697:sgl)
          n399 = Multiply(x=w696, y=w697) -> (x*y=w695:sgl)
          n400 = Divide(x=w695, y=w694) -> (x/y=w693:sgl)
        }
      }
      n401 = case shown="True" w582 {
        tunnel: w568 -> [w705 w712]
        tunnel: w569 -> [w704 w710]
        tunnel: w575 -> [w700 w714]
        tunnel: [w703 w709] -> w581
        tunnel: w570 -> [w699 _]
        frame False {
          # "negative, two's complement"
          n402 = Exclusive Or(1:w699, 2:w700) -> (0:w701:u32)
          n403 = Increment(x=w701) -> (x+1=w706:u32)
          n404 = To Single Precision Float(number=w706) -> (single precision float=w708:sgl)
          n405 = Negate(x=w708) -> (-x=w702:sgl)
          n406 = Multiply(x=w705, y=w702) -> (x*y=w707:sgl)
          n407 = Divide(x=w707, y=w704) -> (x/y=w703:sgl)
        }
        frame True {
          # "positive, straight convert"
          n408 = To Single Precision Float(number=w714) -> (single precision float=w713:sgl)
          n409 = Multiply(x=w712, y=w713) -> (x*y=w711:sgl)
          n410 = Divide(x=w711, y=w710) -> (x/y=w709:sgl)
        }
      }
      n411 = case shown="True" w577 {
        tunnel: w568 -> [w721 w728]
        tunnel: w569 -> [w720 w726]
        tunnel: w574 -> [w716 w730]
        tunnel: [w719 w725] -> w579
        tunnel: w570 -> [w715 _]
        frame False {
          # "negative, two's complement"
          n412 = Exclusive Or(1:w715, 2:w716) -> (0:w717:u32)
          n413 = Increment(x=w717) -> (x+1=w722:u32)
          n414 = To Single Precision Float(number=w722) -> (single precision float=w724:sgl)
          n415 = Negate(x=w724) -> (-x=w718:sgl)
          n416 = Multiply(x=w721, y=w718) -> (x*y=w723:sgl)
          n417 = Divide(x=w723, y=w720) -> (x/y=w719:sgl)
        }
        frame True {
          # "positive, straight convert"
          n418 = To Single Precision Float(number=w730) -> (single precision float=w729:sgl)
          n419 = Multiply(x=w728, y=w729) -> (x*y=w727:sgl)
          n420 = Divide(x=w727, y=w726) -> (x/y=w725:sgl)
        }
      }
      n421 = case shown="True" w576 {
        tunnel: w568 -> [w737 w744]
        tunnel: w569 -> [w736 w742]
        tunnel: w571 -> [w732 w746]
        tunnel: [w735 w741] -> w578
        tunnel: w570 -> [w731 _]
        frame False {
          # "negative, two's complement"
          n422 = Exclusive Or(1:w731, 2:w732) -> (0:w733:u32)
          n423 = Increment(x=w733) -> (x+1=w738:u32)
          n424 = To Single Precision Float(number=w738) -> (single precision float=w740:sgl)
          n425 = Negate(x=w740) -> (-x=w734:sgl)
          n426 = Multiply(x=w737, y=w734) -> (x*y=w739:sgl)
          n427 = Divide(x=w739, y=w736) -> (x/y=w735:sgl)
        }
        frame True {
          # "positive, straight convert"
          n428 = To Single Precision Float(number=w746) -> (single precision float=w745:sgl)
          n429 = Multiply(x=w744, y=w745) -> (x*y=w743:sgl)
          n430 = Divide(x=w743, y=w742) -> (x/y=w741:sgl)
        }
      }
      n431 = case shown="True" w612 {
        tunnel: w568 -> [w753 w760]
        tunnel: w569 -> [w752 w758]
        tunnel: w614 -> [w748 w762]
        tunnel: [w751 w757] -> w613
        tunnel: w570 -> [w747 _]
        frame False {
          # "negative, two's complement"
          n432 = Exclusive Or(1:w747, 2:w748) -> (0:w749:u32)
          n433 = Increment(x=w749) -> (x+1=w754:u32)
          n434 = To Single Precision Float(number=w754) -> (single precision float=w756:sgl)
          n435 = Negate(x=w756) -> (-x=w750:sgl)
          n436 = Multiply(x=w753, y=w750) -> (x*y=w755:sgl)
          n437 = Divide(x=w755, y=w752) -> (x/y=w751:sgl)
        }
        frame True {
          # "positive, straight convert"
          n438 = To Single Precision Float(number=w762) -> (single precision float=w761:sgl)
          n439 = Multiply(x=w760, y=w761) -> (x*y=w759:sgl)
          n440 = Divide(x=w759, y=w758) -> (x/y=w757:sgl)
        }
      }
    }
    frame 16 {
      w783 = u32 262143
      w782 = sgl 131072.0
      w806 = u32 131072
      # "2 ^ 17 for sign bit check"
      # "(2 ^ 18) - 1 for XOR"
      # "Implement NOT(x) as (x XOR ((2 ^ 18) - 1))"
      # "18-bit"
      # "2^17"
      # "data is output as two's complement binary"
      # "if ((a & 0b100000000000000000) == 0) // positive\n      a_ = aRange * float(a) / 131072.0; \n    else // negative\n      a_ = -aRange * float((~a + 1U)) / 131072.0;"
      n441 = String To Byte Array(string=w895) -> (unsigned byte array=w890:u8[])
      n442 = Index Array(array=w890) -> (element #1=w894:u8, element #2=w891:u8, element #3=w882:u8, element #4=w878:u8, element #5=w870:u8, element #6=w865:u8, element #7=w858:u8, element #8=w853:u8, element #9=w849:u8, element #10=w805:u8, element #11=w804:u8, element #12=w803:u8, element #13=w802:u8, element #14=w801:u8, element #15=w800:u8, element #16=w799:u8)  [unwired: 18 in, 2 out]
      n443 = And(x=w882, y=u8 192) -> (x .and. y?=w886:u8)
      n444 = And(x=w882, y=u8 63) -> (x .and. y?=w881:u8)
      n445 = And(x=w870, y=u8 240) -> (x .and. y?=w874:u8)
      n446 = And(x=w870, y=u8 15) -> (x .and. y?=w869:u8)
      n447 = And(x=w858, y=u8 252) -> (x .and. y?=w860:u8)
      n448 = And(x=w858, y=u8 3) -> (x .and. y?=w857:u8)
      n449 = And(x=w803, y=u8 192) -> (x .and. y?=w812:u8)
      n450 = And(x=w803, y=u8 63) -> (x .and. y?=w816:u8)
      n451 = And(x=w801, y=u8 240) -> (x .and. y?=w822:u8)
      n452 = And(x=w801, y=u8 15) -> (x .and. y?=w826:u8)
      n453 = And(x=w799, y=u8 252) -> (x .and. y?=w834:u8)
      n454 = To Unsigned Long Integer(number=w894) -> (unsigned 32bit integer=w889:u32)
      n455 = To Unsigned Long Integer(number=w891) -> (unsigned 32bit integer=w888:u32)
      n456 = To Unsigned Long Integer(number=w886) -> (unsigned 32bit integer=w779:u32)
      n457 = To Unsigned Long Integer(number=w881) -> (unsigned 32bit integer=w880:u32)
      n458 = To Unsigned Long Integer(number=w878) -> (unsigned 32bit integer=w877:u32)
      n459 = To Unsigned Long Integer(number=w874) -> (unsigned 32bit integer=w773:u32)
      n460 = To Unsigned Long Integer(number=w869) -> (unsigned 32bit integer=w867:u32)
      n461 = To Unsigned Long Integer(number=w865) -> (unsigned 32bit integer=w863:u32)
      n462 = To Unsigned Long Integer(number=w860) -> (unsigned 32bit integer=w769:u32)
      n463 = To Unsigned Long Integer(number=w857) -> (unsigned 32bit integer=w855:u32)
      n464 = To Unsigned Long Integer(number=w853) -> (unsigned 32bit integer=w851:u32)
      n465 = To Unsigned Long Integer(number=w849) -> (unsigned 32bit integer=w848:u32)
      n466 = To Unsigned Long Integer(number=w805) -> (unsigned 32bit integer=w809:u32)
      n467 = To Unsigned Long Integer(number=w804) -> (unsigned 32bit integer=w810:u32)
      n468 = To Unsigned Long Integer(number=w812) -> (unsigned 32bit integer=w775:u32)
      n469 = To Unsigned Long Integer(number=w816) -> (unsigned 32bit integer=w817:u32)
      n470 = To Unsigned Long Integer(number=w802) -> (unsigned 32bit integer=w819:u32)
      n471 = To Unsigned Long Integer(number=w822) -> (unsigned 32bit integer=w767:u32)
      n472 = To Unsigned Long Integer(number=w826) -> (unsigned 32bit integer=w828:u32)
      n473 = To Unsigned Long Integer(number=w800) -> (unsigned 32bit integer=w831:u32)
      n474 = To Unsigned Long Integer(number=w834) -> (unsigned 32bit integer=w764:u32)
      n475 = Logical Shift(y=i16 10, x=w889) -> (x << y=w884:u32)
      n476 = Logical Shift(y=i16 2, x=w888) -> (x << y=w885:u32)
      n477 = Logical Shift(y=i16 -6, x=w779) -> (x << y=w778:u32)
      n478 = Logical Shift(y=i16 12, x=w880) -> (x << y=w873:u32)
      n479 = Logical Shift(y=i16 4, x=w877) -> (x << y=w872:u32)
      n480 = Logical Shift(y=i16 -4, x=w773) -> (x << y=w772:u32)
      n481 = Logical Shift(y=i16 14, x=w867) -> (x << y=w866:u32)
      n482 = Logical Shift(y=i16 6, x=w863) -> (x << y=w862:u32)
      n483 = Logical Shift(y=i16 -2, x=w769) -> (x << y=w770:u32)
      n484 = Logical Shift(y=i16 16, x=w855) -> (x << y=w854:u32)
      n485 = Logical Shift(y=i16 8, x=w851) -> (x << y=w850:u32)
      n486 = Logical Shift(y=i16 10, x=w809) -> (x << y=w814:u32)
      n487 = Logical Shift(y=i16 2, x=w810) -> (x << y=w813:u32)
      n488 = Logical Shift(y=i16 -6, x=w775) -> (x << y=w776:u32)
      n489 = Logical Shift(y=i16 12, x=w817) -> (x << y=w823:u32)
      n490 = Logical Shift(y=i16 4, x=w819) -> (x << y=w824:u32)
      n491 = Logical Shift(y=i16 -4, x=w767) -> (x << y=w766:u32)
      n492 = Logical Shift(y=i16 14, x=w828) -> (x << y=w829:u32)
      n493 = Logical Shift(y=i16 6, x=w831) -> (x << y=w832:u32)
      n494 = Logical Shift(y=i16 -2, x=w764) -> (x << y=w763:u32)
      n495 = Compound Arithmetic op=OR(w884, w885, w778) -> (w796:u32)
      n496 = Compound Arithmetic op=OR(w873, w872, w772) -> (w785:u32)
      n497 = Compound Arithmetic op=OR(w866, w862, w770) -> (w788:u32)
      n498 = Compound Arithmetic op=OR(w854, w850, w848) -> (w787:u32)
      n499 = Compound Arithmetic op=OR(w814, w813, w776) -> (w784:u32)
      n500 = Compound Arithmetic op=OR(w823, w824, w766) -> (w842:u32)
      n501 = Compound Arithmetic op=OR(w829, w832, w763) -> (w843:u32)
      n502 = And(x=w806, y=w796) -> (x .and. y?=w847:u32)
      n503 = And(x=w806, y=w785) -> (x .and. y?=w846:u32)
      n504 = And(x=w806, y=w788) -> (x .and. y?=w845:u32)
      n505 = And(x=w806, y=w787) -> (x .and. y?=w844:u32)
      n506 = And(x=w806, y=w784) -> (x .and. y?=w835:u32)
      n507 = And(x=w806, y=w842) -> (x .and. y?=w836:u32)
      n508 = And(x=w806, y=w843) -> (x .and. y?=w837:u32)
      n509 = Equal To 0?(x=w847) -> (x = 0?=w797:bool)
      n510 = Equal To 0?(x=w846) -> (x = 0?=w786:bool)
      n511 = Equal To 0?(x=w845) -> (x = 0?=w795:bool)
      n512 = Equal To 0?(x=w844) -> (x = 0?=w790:bool)
      n513 = Equal To 0?(x=w835) -> (x = 0?=w789:bool)
      n514 = Equal To 0?(x=w836) -> (x = 0?=w838:bool)
      n515 = Equal To 0?(x=w837) -> (x = 0?=w839:bool)
      n516 = case shown="True" w797 {
        tunnel: w781 -> [w902 w909]
        tunnel: w782 -> [w901 w907]
        tunnel: w796 -> [w897 w911]
        tunnel: [w900 w906] -> w798
        tunnel: w783 -> [w896 _]
        frame False {
          # "negative, two's complement"
          n517 = Exclusive Or(1:w896, 2:w897) -> (0:w898:u32)
          n518 = Increment(x=w898) -> (x+1=w903:u32)
          n519 = To Single Precision Float(number=w903) -> (single precision float=w905:sgl)
          n520 = Negate(x=w905) -> (-x=w899:sgl)
          n521 = Multiply(x=w902, y=w899) -> (x*y=w904:sgl)
          n522 = Divide(x=w904, y=w901) -> (x/y=w900:sgl)
        }
        frame True {
          # "positive, straight convert"
          n523 = To Single Precision Float(number=w911) -> (single precision float=w910:sgl)
          n524 = Multiply(x=w909, y=w910) -> (x*y=w908:sgl)
          n525 = Divide(x=w908, y=w907) -> (x/y=w906:sgl)
        }
      }
      n526 = case shown="True" w786 {
        tunnel: w781 -> [w918 w925]
        tunnel: w782 -> [w917 w923]
        tunnel: w785 -> [w913 w927]
        tunnel: [w916 w922] -> w793
        tunnel: w783 -> [w912 _]
        frame False {
          # "negative, two's complement"
          n527 = Exclusive Or(1:w912, 2:w913) -> (0:w914:u32)
          n528 = Increment(x=w914) -> (x+1=w919:u32)
          n529 = To Single Precision Float(number=w919) -> (single precision float=w921:sgl)
          n530 = Negate(x=w921) -> (-x=w915:sgl)
          n531 = Multiply(x=w918, y=w915) -> (x*y=w920:sgl)
          n532 = Divide(x=w920, y=w917) -> (x/y=w916:sgl)
        }
        frame True {
          # "positive, straight convert"
          n533 = To Single Precision Float(number=w927) -> (single precision float=w926:sgl)
          n534 = Multiply(x=w925, y=w926) -> (x*y=w924:sgl)
          n535 = Divide(x=w924, y=w923) -> (x/y=w922:sgl)
        }
      }
      n536 = case shown="True" w795 {
        tunnel: w781 -> [w934 w941]
        tunnel: w782 -> [w933 w939]
        tunnel: w788 -> [w929 w943]
        tunnel: [w932 w938] -> w794
        tunnel: w783 -> [w928 _]
        frame False {
          # "negative, two's complement"
          n537 = Exclusive Or(1:w928, 2:w929) -> (0:w930:u32)
          n538 = Increment(x=w930) -> (x+1=w935:u32)
          n539 = To Single Precision Float(number=w935) -> (single precision float=w937:sgl)
          n540 = Negate(x=w937) -> (-x=w931:sgl)
          n541 = Multiply(x=w934, y=w931) -> (x*y=w936:sgl)
          n542 = Divide(x=w936, y=w933) -> (x/y=w932:sgl)
        }
        frame True {
          # "positive, straight convert"
          n543 = To Single Precision Float(number=w943) -> (single precision float=w942:sgl)
          n544 = Multiply(x=w941, y=w942) -> (x*y=w940:sgl)
          n545 = Divide(x=w940, y=w939) -> (x/y=w938:sgl)
        }
      }
      n546 = case shown="True" w790 {
        tunnel: w781 -> [w950 w957]
        tunnel: w782 -> [w949 w955]
        tunnel: w787 -> [w945 w959]
        tunnel: [w948 w954] -> w792
        tunnel: w783 -> [w944 _]
        frame False {
          # "negative, two's complement"
          n547 = Exclusive Or(1:w944, 2:w945) -> (0:w946:u32)
          n548 = Increment(x=w946) -> (x+1=w951:u32)
          n549 = To Single Precision Float(number=w951) -> (single precision float=w953:sgl)
          n550 = Negate(x=w953) -> (-x=w947:sgl)
          n551 = Multiply(x=w950, y=w947) -> (x*y=w952:sgl)
          n552 = Divide(x=w952, y=w949) -> (x/y=w948:sgl)
        }
        frame True {
          # "positive, straight convert"
          n553 = To Single Precision Float(number=w959) -> (single precision float=w958:sgl)
          n554 = Multiply(x=w957, y=w958) -> (x*y=w956:sgl)
          n555 = Divide(x=w956, y=w955) -> (x/y=w954:sgl)
        }
      }
      n556 = case shown="True" w789 {
        tunnel: w781 -> [w966 w973]
        tunnel: w782 -> [w965 w971]
        tunnel: w784 -> [w961 w975]
        tunnel: [w964 w970] -> w791
        tunnel: w783 -> [w960 _]
        frame False {
          # "negative, two's complement"
          n557 = Exclusive Or(1:w960, 2:w961) -> (0:w962:u32)
          n558 = Increment(x=w962) -> (x+1=w967:u32)
          n559 = To Single Precision Float(number=w967) -> (single precision float=w969:sgl)
          n560 = Negate(x=w969) -> (-x=w963:sgl)
          n561 = Multiply(x=w966, y=w963) -> (x*y=w968:sgl)
          n562 = Divide(x=w968, y=w965) -> (x/y=w964:sgl)
        }
        frame True {
          # "positive, straight convert"
          n563 = To Single Precision Float(number=w975) -> (single precision float=w974:sgl)
          n564 = Multiply(x=w973, y=w974) -> (x*y=w972:sgl)
          n565 = Divide(x=w972, y=w971) -> (x/y=w970:sgl)
        }
      }
      n566 = case shown="True" w838 {
        tunnel: w781 -> [w998 w1005]
        tunnel: w782 -> [w997 w1003]
        tunnel: w842 -> [w993 w1007]
        tunnel: [w996 w1002] -> w840
        tunnel: w783 -> [w992 _]
        frame False {
          # "negative, two's complement"
          n567 = Exclusive Or(1:w992, 2:w993) -> (0:w994:u32)
          n568 = Increment(x=w994) -> (x+1=w999:u32)
          n569 = To Single Precision Float(number=w999) -> (single precision float=w1001:sgl)
          n570 = Negate(x=w1001) -> (-x=w995:sgl)
          n571 = Multiply(x=w998, y=w995) -> (x*y=w1000:sgl)
          n572 = Divide(x=w1000, y=w997) -> (x/y=w996:sgl)
        }
        frame True {
          # "positive, straight convert"
          n573 = To Single Precision Float(number=w1007) -> (single precision float=w1006:sgl)
          n574 = Multiply(x=w1005, y=w1006) -> (x*y=w1004:sgl)
          n575 = Divide(x=w1004, y=w1003) -> (x/y=w1002:sgl)
        }
      }
      n576 = case shown="True" w839 {
        tunnel: w781 -> [w982 w989]
        tunnel: w782 -> [w981 w987]
        tunnel: w843 -> [w977 w991]
        tunnel: [w980 w986] -> w841
        tunnel: w783 -> [w976 _]
        frame False {
          # "negative, two's complement"
          n577 = Exclusive Or(1:w976, 2:w977) -> (0:w978:u32)
          n578 = Increment(x=w978) -> (x+1=w983:u32)
          n579 = To Single Precision Float(number=w983) -> (single precision float=w985:sgl)
          n580 = Negate(x=w985) -> (-x=w979:sgl)
          n581 = Multiply(x=w982, y=w979) -> (x*y=w984:sgl)
          n582 = Divide(x=w984, y=w981) -> (x/y=w980:sgl)
        }
        frame True {
          # "positive, straight convert"
          n583 = To Single Precision Float(number=w991) -> (single precision float=w990:sgl)
          n584 = Multiply(x=w989, y=w990) -> (x*y=w988:sgl)
          n585 = Divide(x=w988, y=w987) -> (x/y=w986:sgl)
        }
      }
    }
    frame 18, Default {
      w1028 = u32 262143
      w1027 = sgl 131072.0
      w1056 = u32 131072
      # "2 ^ 17 for sign bit check"
      # "(2 ^ 18) - 1 for XOR"
      # "Implement NOT(x) as (x XOR ((2 ^ 18) - 1))"
      # "18-bit"
      # "2^17"
      # "data is output as two's complement binary"
      # "if ((a & 0b100000000000000000) == 0) // positive\n      a_ = aRange * float(a) / 131072.0; \n    else // negative\n      a_ = -aRange * float((~a + 1U)) / 131072.0;"
      n586 = String To Byte Array(string=w1155) -> (unsigned byte array=w1150:u8[])
      n587 = Index Array(array=w1150) -> (element #1=w1154:u8, element #2=w1151:u8, element #3=w1142:u8, element #4=w1138:u8, element #5=w1130:u8, element #6=w1125:u8, element #7=w1118:u8, element #8=w1113:u8, element #9=w1109:u8, element #10=w1055:u8, element #11=w1054:u8, element #12=w1053:u8, element #13=w1052:u8, element #14=w1051:u8, element #15=w1050:u8, element #16=w1049:u8, element #17=w1048:u8, element #18=w1047:u8)  [unwired: 18 in]
      n588 = And(x=w1142, y=u8 192) -> (x .and. y?=w1146:u8)
      n589 = And(x=w1142, y=u8 63) -> (x .and. y?=w1141:u8)
      n590 = And(x=w1130, y=u8 240) -> (x .and. y?=w1134:u8)
      n591 = And(x=w1130, y=u8 15) -> (x .and. y?=w1129:u8)
      n592 = And(x=w1118, y=u8 252) -> (x .and. y?=w1120:u8)
      n593 = And(x=w1118, y=u8 3) -> (x .and. y?=w1117:u8)
      n594 = And(x=w1053, y=u8 192) -> (x .and. y?=w1062:u8)
      n595 = And(x=w1053, y=u8 63) -> (x .and. y?=w1066:u8)
      n596 = And(x=w1051, y=u8 240) -> (x .and. y?=w1072:u8)
      n597 = And(x=w1051, y=u8 15) -> (x .and. y?=w1076:u8)
      n598 = And(x=w1049, y=u8 252) -> (x .and. y?=w1084:u8)
      n599 = And(x=w1049, y=u8 3) -> (x .and. y?=w1086:u8)
      n600 = To Unsigned Long Integer(number=w1154) -> (unsigned 32bit integer=w1149:u32)
      n601 = To Unsigned Long Integer(number=w1151) -> (unsigned 32bit integer=w1148:u32)
      n602 = To Unsigned Long Integer(number=w1146) -> (unsigned 32bit integer=w1024:u32)
      n603 = To Unsigned Long Integer(number=w1141) -> (unsigned 32bit integer=w1140:u32)
      n604 = To Unsigned Long Integer(number=w1138) -> (unsigned 32bit integer=w1137:u32)
      n605 = To Unsigned Long Integer(number=w1134) -> (unsigned 32bit integer=w1018:u32)
      n606 = To Unsigned Long Integer(number=w1129) -> (unsigned 32bit integer=w1127:u32)
      n607 = To Unsigned Long Integer(number=w1125) -> (unsigned 32bit integer=w1123:u32)
      n608 = To Unsigned Long Integer(number=w1120) -> (unsigned 32bit integer=w1014:u32)
      n609 = To Unsigned Long Integer(number=w1117) -> (unsigned 32bit integer=w1115:u32)
      n610 = To Unsigned Long Integer(number=w1113) -> (unsigned 32bit integer=w1111:u32)
      n611 = To Unsigned Long Integer(number=w1109) -> (unsigned 32bit integer=w1108:u32)
      n612 = To Unsigned Long Integer(number=w1055) -> (unsigned 32bit integer=w1059:u32)
      n613 = To Unsigned Long Integer(number=w1054) -> (unsigned 32bit integer=w1060:u32)
      n614 = To Unsigned Long Integer(number=w1062) -> (unsigned 32bit integer=w1020:u32)
      n615 = To Unsigned Long Integer(number=w1066) -> (unsigned 32bit integer=w1067:u32)
      n616 = To Unsigned Long Integer(number=w1052) -> (unsigned 32bit integer=w1069:u32)
      n617 = To Unsigned Long Integer(number=w1072) -> (unsigned 32bit integer=w1012:u32)
      n618 = To Unsigned Long Integer(number=w1076) -> (unsigned 32bit integer=w1078:u32)
      n619 = To Unsigned Long Integer(number=w1050) -> (unsigned 32bit integer=w1081:u32)
      n620 = To Unsigned Long Integer(number=w1084) -> (unsigned 32bit integer=w1009:u32)
      n621 = To Unsigned Long Integer(number=w1086) -> (unsigned 32bit integer=w1088:u32)
      n622 = To Unsigned Long Integer(number=w1048) -> (unsigned 32bit integer=w1091:u32)
      n623 = To Unsigned Long Integer(number=w1047) -> (unsigned 32bit integer=w1093:u32)
      n624 = Logical Shift(y=i16 10, x=w1149) -> (x << y=w1144:u32)
      n625 = Logical Shift(y=i16 2, x=w1148) -> (x << y=w1145:u32)
      n626 = Logical Shift(y=i16 -6, x=w1024) -> (x << y=w1023:u32)
      n627 = Logical Shift(y=i16 12, x=w1140) -> (x << y=w1133:u32)
      n628 = Logical Shift(y=i16 4, x=w1137) -> (x << y=w1132:u32)
      n629 = Logical Shift(y=i16 -4, x=w1018) -> (x << y=w1017:u32)
      n630 = Logical Shift(y=i16 14, x=w1127) -> (x << y=w1126:u32)
      n631 = Logical Shift(y=i16 6, x=w1123) -> (x << y=w1122:u32)
      n632 = Logical Shift(y=i16 -2, x=w1014) -> (x << y=w1015:u32)
      n633 = Logical Shift(y=i16 16, x=w1115) -> (x << y=w1114:u32)
      n634 = Logical Shift(y=i16 8, x=w1111) -> (x << y=w1110:u32)
      n635 = Logical Shift(y=i16 10, x=w1059) -> (x << y=w1064:u32)
      n636 = Logical Shift(y=i16 2, x=w1060) -> (x << y=w1063:u32)
      n637 = Logical Shift(y=i16 -6, x=w1020) -> (x << y=w1021:u32)
      n638 = Logical Shift(y=i16 12, x=w1067) -> (x << y=w1073:u32)
      n639 = Logical Shift(y=i16 4, x=w1069) -> (x << y=w1074:u32)
      n640 = Logical Shift(y=i16 -4, x=w1012) -> (x << y=w1011:u32)
      n641 = Logical Shift(y=i16 14, x=w1078) -> (x << y=w1079:u32)
      n642 = Logical Shift(y=i16 6, x=w1081) -> (x << y=w1082:u32)
      n643 = Logical Shift(y=i16 -2, x=w1009) -> (x << y=w1008:u32)
      n644 = Logical Shift(y=i16 16, x=w1088) -> (x << y=w1089:u32)
      n645 = Logical Shift(y=i16 8, x=w1091) -> (x << y=w1092:u32)
      n646 = Compound Arithmetic op=OR(w1144, w1145, w1023) -> (w1041:u32)
      n647 = Compound Arithmetic op=OR(w1133, w1132, w1017) -> (w1030:u32)
      n648 = Compound Arithmetic op=OR(w1126, w1122, w1015) -> (w1033:u32)
      n649 = Compound Arithmetic op=OR(w1114, w1110, w1108) -> (w1032:u32)
      n650 = Compound Arithmetic op=OR(w1064, w1063, w1021) -> (w1029:u32)
      n651 = Compound Arithmetic op=OR(w1073, w1074, w1011) -> (w1102:u32)
      n652 = Compound Arithmetic op=OR(w1079, w1082, w1008) -> (w1103:u32)
      n653 = Compound Arithmetic op=OR(w1089, w1092, w1093) -> (w1046:u32)
      n654 = And(x=w1056, y=w1041) -> (x .and. y?=w1107:u32)
      n655 = And(x=w1056, y=w1030) -> (x .and. y?=w1106:u32)
      n656 = And(x=w1056, y=w1033) -> (x .and. y?=w1105:u32)
      n657 = And(x=w1056, y=w1032) -> (x .and. y?=w1104:u32)
      n658 = And(x=w1056, y=w1029) -> (x .and. y?=w1094:u32)
      n659 = And(x=w1056, y=w1102) -> (x .and. y?=w1095:u32)
      n660 = And(x=w1056, y=w1103) -> (x .and. y?=w1096:u32)
      n661 = And(x=w1056, y=w1046) -> (x .and. y?=w1101:u32)
      n662 = Equal To 0?(x=w1107) -> (x = 0?=w1042:bool)
      n663 = Equal To 0?(x=w1106) -> (x = 0?=w1031:bool)
      n664 = Equal To 0?(x=w1105) -> (x = 0?=w1040:bool)
      n665 = Equal To 0?(x=w1104) -> (x = 0?=w1035:bool)
      n666 = Equal To 0?(x=w1094) -> (x = 0?=w1034:bool)
      n667 = Equal To 0?(x=w1095) -> (x = 0?=w1097:bool)
      n668 = Equal To 0?(x=w1096) -> (x = 0?=w1098:bool)
      n669 = Equal To 0?(x=w1101) -> (x = 0?=w1045:bool)
      n670 = case shown="True" w1042 {
        tunnel: w1026 -> [w1162 w1169]
        tunnel: w1027 -> [w1161 w1167]
        tunnel: w1041 -> [w1157 w1171]
        tunnel: [w1160 w1166] -> w1043
        tunnel: w1028 -> [w1156 _]
        frame False {
          # "negative, two's complement"
          n671 = Exclusive Or(1:w1156, 2:w1157) -> (0:w1158:u32)
          n672 = Increment(x=w1158) -> (x+1=w1163:u32)
          n673 = To Single Precision Float(number=w1163) -> (single precision float=w1165:sgl)
          n674 = Negate(x=w1165) -> (-x=w1159:sgl)
          n675 = Multiply(x=w1162, y=w1159) -> (x*y=w1164:sgl)
          n676 = Divide(x=w1164, y=w1161) -> (x/y=w1160:sgl)
        }
        frame True {
          # "positive, straight convert"
          n677 = To Single Precision Float(number=w1171) -> (single precision float=w1170:sgl)
          n678 = Multiply(x=w1169, y=w1170) -> (x*y=w1168:sgl)
          n679 = Divide(x=w1168, y=w1167) -> (x/y=w1166:sgl)
        }
      }
      n680 = case shown="True" w1031 {
        tunnel: w1026 -> [w1178 w1185]
        tunnel: w1027 -> [w1177 w1183]
        tunnel: w1030 -> [w1173 w1187]
        tunnel: [w1176 w1182] -> w1038
        tunnel: w1028 -> [w1172 _]
        frame False {
          # "negative, two's complement"
          n681 = Exclusive Or(1:w1172, 2:w1173) -> (0:w1174:u32)
          n682 = Increment(x=w1174) -> (x+1=w1179:u32)
          n683 = To Single Precision Float(number=w1179) -> (single precision float=w1181:sgl)
          n684 = Negate(x=w1181) -> (-x=w1175:sgl)
          n685 = Multiply(x=w1178, y=w1175) -> (x*y=w1180:sgl)
          n686 = Divide(x=w1180, y=w1177) -> (x/y=w1176:sgl)
        }
        frame True {
          # "positive, straight convert"
          n687 = To Single Precision Float(number=w1187) -> (single precision float=w1186:sgl)
          n688 = Multiply(x=w1185, y=w1186) -> (x*y=w1184:sgl)
          n689 = Divide(x=w1184, y=w1183) -> (x/y=w1182:sgl)
        }
      }
      n690 = case shown="True" w1040 {
        tunnel: w1026 -> [w1194 w1201]
        tunnel: w1027 -> [w1193 w1199]
        tunnel: w1033 -> [w1189 w1203]
        tunnel: [w1192 w1198] -> w1039
        tunnel: w1028 -> [w1188 _]
        frame False {
          # "negative, two's complement"
          n691 = Exclusive Or(1:w1188, 2:w1189) -> (0:w1190:u32)
          n692 = Increment(x=w1190) -> (x+1=w1195:u32)
          n693 = To Single Precision Float(number=w1195) -> (single precision float=w1197:sgl)
          n694 = Negate(x=w1197) -> (-x=w1191:sgl)
          n695 = Multiply(x=w1194, y=w1191) -> (x*y=w1196:sgl)
          n696 = Divide(x=w1196, y=w1193) -> (x/y=w1192:sgl)
        }
        frame True {
          # "positive, straight convert"
          n697 = To Single Precision Float(number=w1203) -> (single precision float=w1202:sgl)
          n698 = Multiply(x=w1201, y=w1202) -> (x*y=w1200:sgl)
          n699 = Divide(x=w1200, y=w1199) -> (x/y=w1198:sgl)
        }
      }
      n700 = case shown="True" w1035 {
        tunnel: w1026 -> [w1210 w1217]
        tunnel: w1027 -> [w1209 w1215]
        tunnel: w1032 -> [w1205 w1219]
        tunnel: [w1208 w1214] -> w1037
        tunnel: w1028 -> [w1204 _]
        frame False {
          # "negative, two's complement"
          n701 = Exclusive Or(1:w1204, 2:w1205) -> (0:w1206:u32)
          n702 = Increment(x=w1206) -> (x+1=w1211:u32)
          n703 = To Single Precision Float(number=w1211) -> (single precision float=w1213:sgl)
          n704 = Negate(x=w1213) -> (-x=w1207:sgl)
          n705 = Multiply(x=w1210, y=w1207) -> (x*y=w1212:sgl)
          n706 = Divide(x=w1212, y=w1209) -> (x/y=w1208:sgl)
        }
        frame True {
          # "positive, straight convert"
          n707 = To Single Precision Float(number=w1219) -> (single precision float=w1218:sgl)
          n708 = Multiply(x=w1217, y=w1218) -> (x*y=w1216:sgl)
          n709 = Divide(x=w1216, y=w1215) -> (x/y=w1214:sgl)
        }
      }
      n710 = case shown="True" w1034 {
        tunnel: w1026 -> [w1226 w1233]
        tunnel: w1027 -> [w1225 w1231]
        tunnel: w1029 -> [w1221 w1235]
        tunnel: [w1224 w1230] -> w1036
        tunnel: w1028 -> [w1220 _]
        frame False {
          # "negative, two's complement"
          n711 = Exclusive Or(1:w1220, 2:w1221) -> (0:w1222:u32)
          n712 = Increment(x=w1222) -> (x+1=w1227:u32)
          n713 = To Single Precision Float(number=w1227) -> (single precision float=w1229:sgl)
          n714 = Negate(x=w1229) -> (-x=w1223:sgl)
          n715 = Multiply(x=w1226, y=w1223) -> (x*y=w1228:sgl)
          n716 = Divide(x=w1228, y=w1225) -> (x/y=w1224:sgl)
        }
        frame True {
          # "positive, straight convert"
          n717 = To Single Precision Float(number=w1235) -> (single precision float=w1234:sgl)
          n718 = Multiply(x=w1233, y=w1234) -> (x*y=w1232:sgl)
          n719 = Divide(x=w1232, y=w1231) -> (x/y=w1230:sgl)
        }
      }
      n720 = case shown="True" w1097 {
        tunnel: w1026 -> [w1274 w1281]
        tunnel: w1027 -> [w1273 w1279]
        tunnel: w1102 -> [w1269 w1283]
        tunnel: [w1272 w1278] -> w1099
        tunnel: w1028 -> [w1268 _]
        frame False {
          # "negative, two's complement"
          n721 = Exclusive Or(1:w1268, 2:w1269) -> (0:w1270:u32)
          n722 = Increment(x=w1270) -> (x+1=w1275:u32)
          n723 = To Single Precision Float(number=w1275) -> (single precision float=w1277:sgl)
          n724 = Negate(x=w1277) -> (-x=w1271:sgl)
          n725 = Multiply(x=w1274, y=w1271) -> (x*y=w1276:sgl)
          n726 = Divide(x=w1276, y=w1273) -> (x/y=w1272:sgl)
        }
        frame True {
          # "positive, straight convert"
          n727 = To Single Precision Float(number=w1283) -> (single precision float=w1282:sgl)
          n728 = Multiply(x=w1281, y=w1282) -> (x*y=w1280:sgl)
          n729 = Divide(x=w1280, y=w1279) -> (x/y=w1278:sgl)
        }
      }
      n730 = case shown="True" w1098 {
        tunnel: w1026 -> [w1258 w1265]
        tunnel: w1027 -> [w1257 w1263]
        tunnel: w1103 -> [w1253 w1267]
        tunnel: [w1256 w1262] -> w1100
        tunnel: w1028 -> [w1252 _]
        frame False {
          # "negative, two's complement"
          n731 = Exclusive Or(1:w1252, 2:w1253) -> (0:w1254:u32)
          n732 = Increment(x=w1254) -> (x+1=w1259:u32)
          n733 = To Single Precision Float(number=w1259) -> (single precision float=w1261:sgl)
          n734 = Negate(x=w1261) -> (-x=w1255:sgl)
          n735 = Multiply(x=w1258, y=w1255) -> (x*y=w1260:sgl)
          n736 = Divide(x=w1260, y=w1257) -> (x/y=w1256:sgl)
        }
        frame True {
          # "positive, straight convert"
          n737 = To Single Precision Float(number=w1267) -> (single precision float=w1266:sgl)
          n738 = Multiply(x=w1265, y=w1266) -> (x*y=w1264:sgl)
          n739 = Divide(x=w1264, y=w1263) -> (x/y=w1262:sgl)
        }
      }
      n740 = case shown="True" w1045 {
        tunnel: w1026 -> [w1242 w1249]
        tunnel: w1027 -> [w1241 w1247]
        tunnel: w1046 -> [w1237 w1251]
        tunnel: [w1240 w1246] -> w1044
        tunnel: w1028 -> [w1236 _]
        frame False {
          # "negative, two's complement"
          n741 = Exclusive Or(1:w1236, 2:w1237) -> (0:w1238:u32)
          n742 = Increment(x=w1238) -> (x+1=w1243:u32)
          n743 = To Single Precision Float(number=w1243) -> (single precision float=w1245:sgl)
          n744 = Negate(x=w1245) -> (-x=w1239:sgl)
          n745 = Multiply(x=w1242, y=w1239) -> (x*y=w1244:sgl)
          n746 = Divide(x=w1244, y=w1241) -> (x/y=w1240:sgl)
        }
        frame True {
          # "positive, straight convert"
          n747 = To Single Precision Float(number=w1251) -> (single precision float=w1250:sgl)
          n748 = Multiply(x=w1249, y=w1250) -> (x*y=w1248:sgl)
          n749 = Divide(x=w1248, y=w1247) -> (x/y=w1246:sgl)
        }
      }
    }
  }
  "V1 (V)" <- w7
  "V2 (V)" <- w5
  "V3 (V)" <- w6
  "V4 (V)" <- w4
  "V5 (V)" <- w3
  "V6 (V)" <- w9
  "V7 (V)" <- w10
  "V8 (V)" <- w8
